vi "TestInitializeLocalLogMultipleSinksAdded_MultipleValidSinkRefsReturned.vi"(8 "error in (no error)":errorcluster, 11 "TestCase in":refnum<class "TestMalleableInterface.lvclass">) -> (0 "error out":errorcluster, 3 "TestCase out":refnum<class "TestMalleableInterface.lvclass">)   [LabVIEW 2017, in "TestMalleableInterface.lvclass"]
uses:
  TestMalleableInterface.lvclass
  Source/Composed Log/LoggerReference/LoggerReference.lvclass/LoggerReference.ctl
  8d299841-f253-422a-a7a1-59edf70c310f.vi
  Source/Composed Log/LoggerReference/Return Aggregate Queues.vi
  Source/Composed Log/LoggerReference/Add Aggregate Log.vi
  8d299841-f253-422a-a7a1-59edf70c310f.vi/5b0dd9e9-b1f9-4760-9dae-818d6c719326.vi
  Source/Composed Log/LoggerReference/Send Add Sink.vi
  Source/LVQueue Sink/LVQueue Sink.lvclass
  C:/CS/Internal/LabVIEW/Logger/Source/Composed Log/Log Sink/Log Sink.lvclass
  Source/Composed Log/Application Logger/Launch Worker Loop.vi
  Source/Composed Log/LoggerReference/Initialize Logger Instance.vi
  Source/Composed Log/LoggerReference/LoggerReference.lvclass
  Source/Composed Log/IErrorFormat/IErrorFormat.lvclass
  Source/Composed Log/Log Sink/Log Sink.lvclass
  <vilib>/addons/_JKI Toolkits/VI Tester/TestCase.llb/TestCase.lvclass
  C:/Program Files (x86)/National Instruments/LabVIEW 2017/vi.lib/addons/_JKI Toolkits/VI Tester/TestCase.llb/TestCase.lvclass
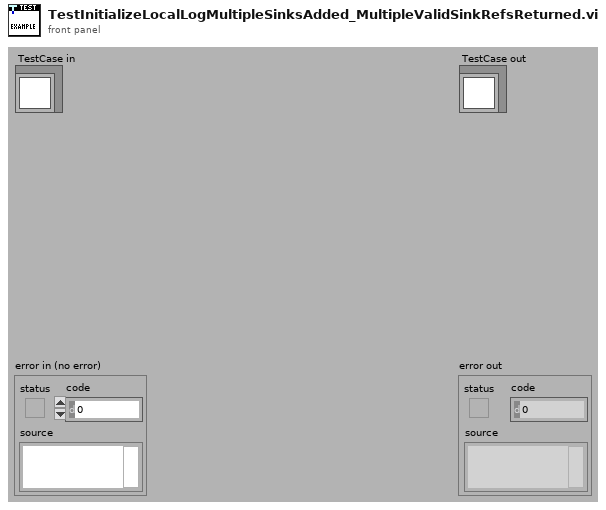
[diagram p1: front panel]
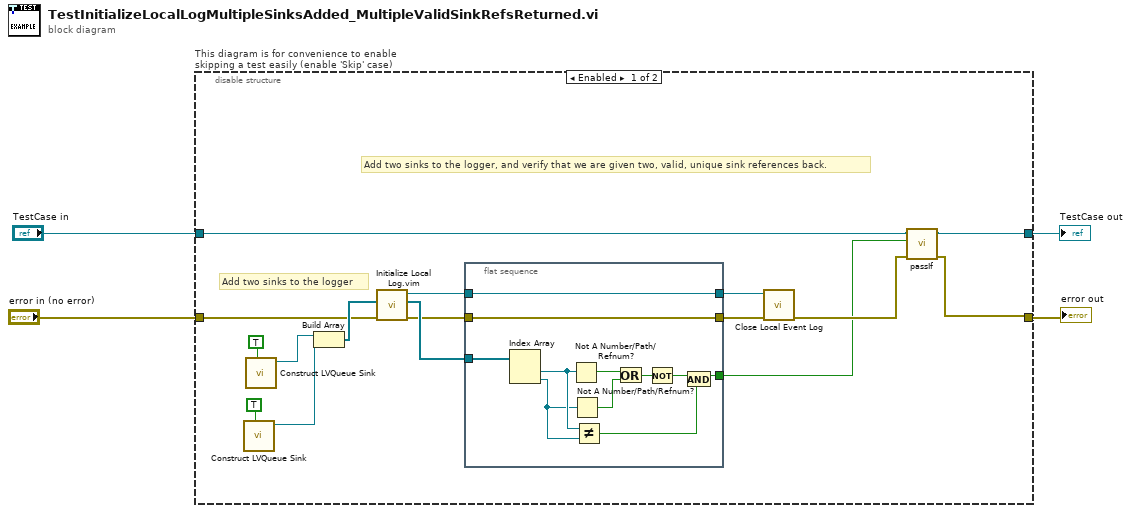
[diagram p0: block diagram]
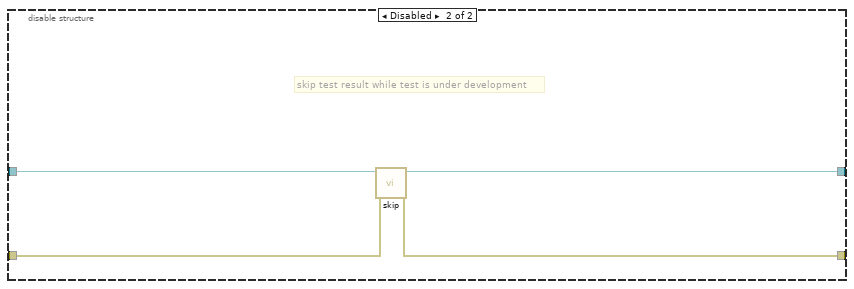
[diagram p2: hidden frame]
diagram:
  n1 = disable-structure "This diagram is for convenience to enable skipping a test easily (enable 'Skip' case)" shown="Enabled" {
    disable-tunnel: "TestCase in" -> [w11 w35]
    disable-tunnel: [w12 w33] -> w1
    disable-tunnel: [w13 w34] -> w3
    disable-tunnel: "error in (no error)" -> [w17 w32]
    frame Enabled {
      # "Add two sinks to the logger, and verify that we are given two, valid, unique sink references back."
      # "Add two sinks to the logger"
      n2 = call "Construct LVQueue Sink.vi"("User Shutdown? (F)"=TRUE) -> ("LVQueue Sink out"=w15:refnum<class "LVQueue Sink.lvclass">)  [unwired: 9 in, 1 out]
      n3 = call "Construct LVQueue Sink.vi"("User Shutdown? (F)"=TRUE) -> ("LVQueue Sink out"=w16:refnum<class "LVQueue Sink.lvclass">)  [unwired: 9 in, 1 out]
      n4 = Build Array(w16, w15) -> (w18:refnum<class "LVQueue Sink.lvclass">[])
      n5 = call "Initialize Local Log.vim"("error in (no error)"=w17, "Startup Sink(s)"=w18) -> ("error out"=w7:errorcluster, "Log Sink Reference(s)"=w10:refnum<data-value>[], "Log Instance Reference"=w8:refnum<class "LoggerReference.lvclass">)  [unwired: 7 in]
      n6 = flat-sequence {
        tunnel: w10 -> [w31]
        tunnel: [w22] -> w9
        tunnel: w8 -> [w26]
        tunnel: w7 -> [w25]
        tunnel: [w26] -> w6
        tunnel: [w25] -> w5
        frame #0 {
          n7 = Index Array(array=w31) -> (element #1=w24:refnum<data-value>, element #2=w23:refnum<data-value>)  [unwired: 2 in]
          n8 = Not A Number/Path/Refnum?(number/path/refnum=w24) -> (NaN/Path/Refnum?=w30:bool)
          n9 = Not A Number/Path/Refnum?(number/path/refnum=w23) -> (NaN/Path/Refnum?=w29:bool)
          n10 = Not Equal?(x=w24, y=w23) -> (x != y?=w21:bool)
          n11 = Or(x=w30, y=w29) -> (x .or. y?=w28:bool)
          n12 = Not(x=w28) -> (.not. x?=w27:bool)
          n13 = And(x=w27, y=w21) -> (x .and. y?=w22:bool)
        }
      }
      n14 = call "Close Local Event Log.vi"("error in (no error)"=w5, "Log Instance"=w6) -> ("error out"=w14:errorcluster)  [unwired: 9 in]
      n15 = call-dynamic "passIf.vi"("error in (no error)"=w14, "pass"=w9, "TestCase in"=w11) -> ("error out"=w13:errorcluster, "TestCase out"=w12:refnum<class "TestMalleableInterface.lvclass">)  [unwired: 7 in]
    }
    frame Disabled {
      # "skip test result while test is under development"
      n16 = call <vilib>:"skip.vi"("error in (no error)"=w32, "TestCase in"=w35) -> ("error out"=w34:errorcluster, "TestCase out"=w33:refnum<class "TestMalleableInterface.lvclass">)  [unwired: 8 in]
    }
  }
  "error out" <- w3
  "TestCase out" <- w1
